vi "Pressure Temperature Monitor.vi"() -> ()   [LabVIEW 2016]
panel:
  in  "Gain":dbl=-10.0 format="%#_13g"
  out "Tempreture":dbl=48.010835359905556 format="%.1f"
  out "Pressure":dbl=1.1830275556146258e-06 format="%#.2e"
  out "Sample Tempreture":dbl(graph)=48.010835359905556
  in  "?":bool
  out "Overdosing":bool
  in  "Dosing Limit":dbl=20.0 format="%#.2f"
  in  "Base Pressure":dbl=6.47 format="%#.2e"
  out "Pressure":dbl(graph)=1.1830275556146258e-06
  out "L":dbl format="%.1f"
  in  "Pressure Limit":dbl=10.0 format="%#.2e"
  in  "?":bool
  # "Pressure (Torr)"
  # "Temperature (°C )"
  # "Langmuir"
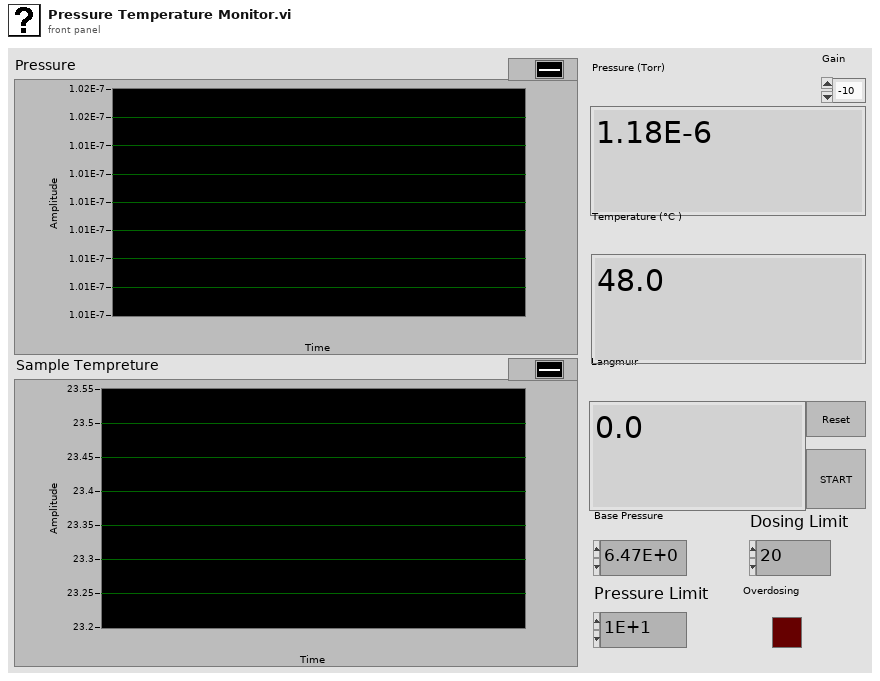
[diagram p1: front panel]
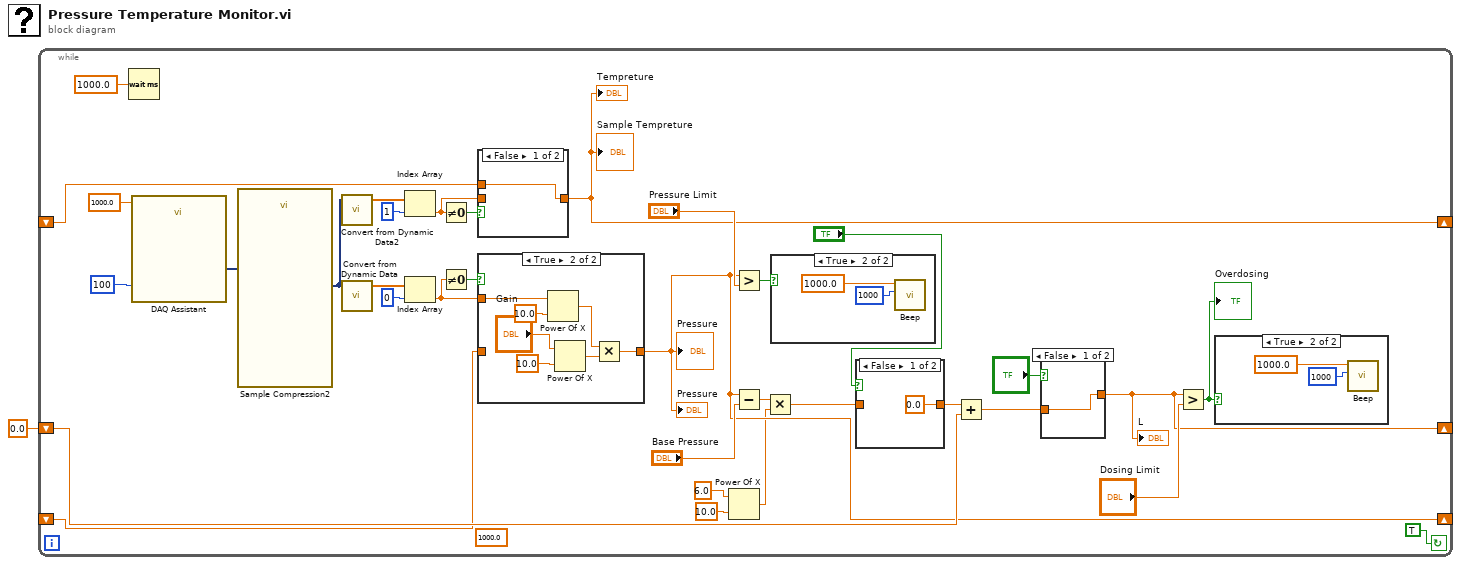
[diagram p0: block diagram]
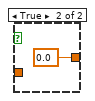
[diagram p4: hidden frame]
diagram:
  n1 = while {
    shift-left: 0.0 -> [w26]
    shift-right: [w24] -> _
    shift-right: [w12] -> _
    shift-left: _ -> [w13]
    shift-right: [w10] -> _
    shift-left: _ -> [w17]
    stop <- TRUE continue-if-true
    (unwired) 1000.0 ("rate")
    n2 = Wait (ms)(milliseconds to wait=1000.0 ("y")) -> ()  [unwired: 1 out]
    n3 = call "DAQ Assistant"("rate"=1000.0, "number of samples"=100) -> ("data"=w2:dynamicdata)  [unwired: 15 in, 2 out]
    n4 = call "Sample Compression2"("Signals"=w2) -> ("Mean"=w18:dynamicdata)  [unwired: 8 in, 2 out]
    n5 = call "Convert from Dynamic Data2"("Dynamic Data Type"=w18) -> ("Array"=w20:dbl[])  [unwired: 3 in]
    n6 = call "Convert from Dynamic Data"("Dynamic Data Type"=w18) -> ("Array"=w22:dbl[])  [unwired: 3 in]
    n7 = Index Array(array=w20, index=1) -> (element=w16:dbl)
    n8 = Index Array(array=w22, index=0) -> (element=w14:dbl)
    n9 = Not Equal To 0?(x=w16) -> (x != 0?=w15:bool)
    n10 = Not Equal To 0?(x=w14) -> (x != 0?=w11:bool)
    n11 = case shown="False" w15 {
      tunnel: w16 -> [_ w45]
      tunnel: [w44 w45] -> w10
      tunnel: w17 -> [w44 _]
      frame False {
      }
      frame True {
      }
    }
    "Sample Tempreture" <- w10
    "Tempreture" <- w10
    n12 = case shown="True" w11 {
      tunnel: w14 -> [_ w42]
      tunnel: [w36 w43] -> w12
      tunnel: w13 -> [w36 _]
      frame False {
      }
      frame True {
        n13 = Power Of X(1:10.0 ("x"), 2:w42) -> (0:w41:dbl)
        n14 = Power Of X(1:10.0 ("x"), 2:"Gain") -> (0:w39:dbl)
        n15 = Multiply(x=w41, y=w39) -> (x*y=w43:dbl)
      }
    }
    "Pressure" <- w12
    "Pressure" <- w12
    n16 = Power Of X(1:10.0 ("x"), 2:6.0 ("y")) -> (0:w6:dbl)
    n17 = Greater?(x=w12, y="Pressure Limit") -> (0:w34:bool)
    n18 = Subtract(x=w12, y="Base Pressure") -> (x-y=w9:dbl)
    n19 = Multiply(x=w9, y=w6) -> (x*y=w5:dbl)
    n20 = case shown="True" w34 {
      frame False {
      }
      frame True {
        n21 = call <vilib>:"Beep.vi"("duration (msec)"=i16 1000 ("duration (msec) - ignored"), "frequency (Hz)"=1000.0 ("frequency (Hz) - ignored")) -> ()  [unwired: 10 in]
      }
    }
    n22 = case shown="False" "?" {
      tunnel: [0.0 w51] -> w27
      tunnel: w5 -> [_ w51]
      frame False {
      }
      frame True {
      }
    }
    n23 = Add(x=w27, y=w26) -> (x+y=w25:dbl)
    n24 = case shown="False" "?" {
      tunnel: w25 -> [w46 _]
      tunnel: [w46 0.0 ("y")] -> w24
      frame False {
      }
      frame True {
      }
    }
    "L" <- w24
    n25 = Greater?(x=w24, y="Dosing Limit") -> (0:w28:bool)
    "Overdosing" <- w28
    n26 = case shown="True" w28 {
      frame False {
      }
      frame True {
        n27 = call <vilib>:"Beep.vi"("duration (msec)"=i16 1000 ("duration (msec) - ignored"), "frequency (Hz)"=1000.0 ("frequency (Hz) - ignored")) -> ()  [unwired: 10 in]
      }
    }
  }
